vi "创建demo守护脚本文件.vi"(8 "错误输入":errorcluster, 11 "文件路径（使用对话框）":path) -> (0 "错误输出":errorcluster)   [LabVIEW 2016]
panel:
  out "连接的字符串":string
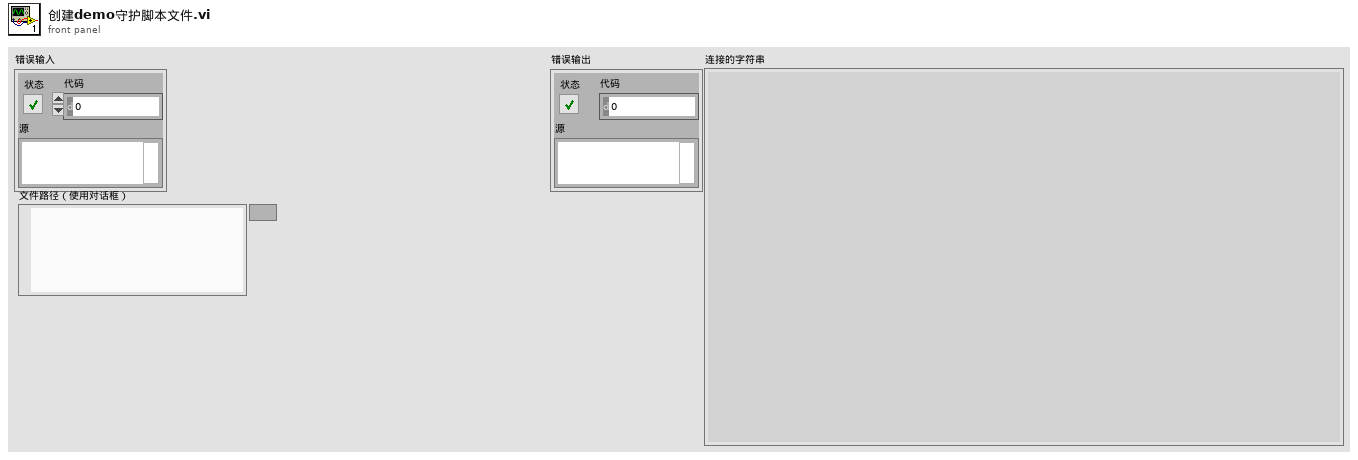
[diagram p1: front panel]
types:
  T1 = enum16{"open", "replace", "create", "open or create", "replace or create", "replace or create with confirmation"}
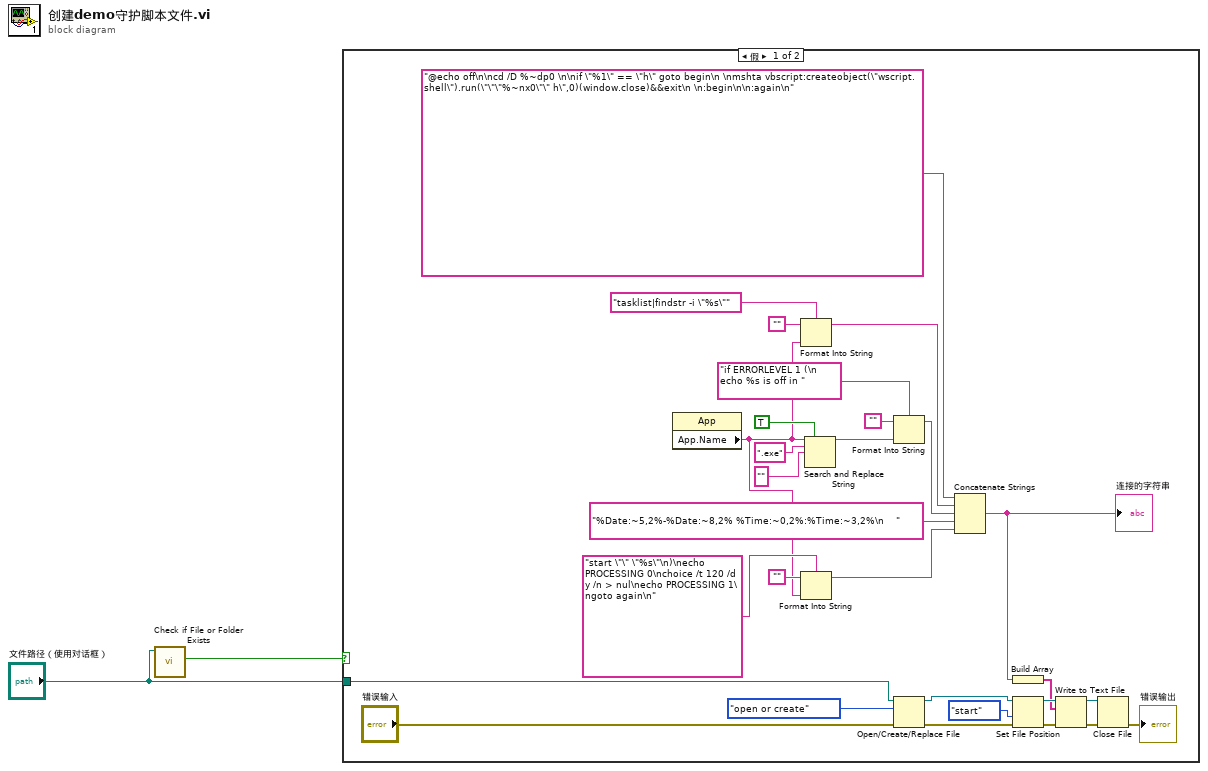
[diagram p0: block diagram]
diagram:
  n1 = call <vilib>:"Check if File or Folder Exists.vi"("path"="文件路径（使用对话框）") -> ("file or folder exists?"=w1:bool)  [unwired: 8 in, 2 out]
  n2 = case shown="假" w1 {
    tunnel: "文件路径（使用对话框）" -> [w3 _]
    frame False {
      n3 = property class="App"() -> ("App.Name"=w6:string)  [unwired: 2 in, 2 out]
      n4 = Format Into String(format string="tasklist|findstr -i \"%s\"", initial string="", w6) -> (resulting string=w10:string)  [unwired: 1 in, 1 out]
      n5 = Format Into String(format string="start \"\" \"%s\"\n)\necho PROCESSING 0\nchoice /t 120 /d y /n > nul\necho PROCESSING 1\ngoto again\n", initial string="", w6) -> (resulting string=w4:string)  [unwired: 1 in, 1 out]
      n6 = Search and Replace String(replace all?=TRUE ("替换全部？(F)"), input string=w6, search string=".exe" ("搜索字符串"), replace string="" ("替换字符串(\"\")")) -> (result string=w12:string)  [unwired: 4 in, 3 out]
      n7 = Format Into String(format string="if ERRORLEVEL 1 (\n    echo %s is off in ", initial string="", w12) -> (resulting string=w9:string)  [unwired: 1 in, 1 out]
      n8 = Open/Create/Replace File(file path (use dialog)=w3, error in="错误输入", operation (0:open)=T1."open or create" ("操作(0:open)")) -> (refnum out=w27:refnum<file>, error out=w28:errorcluster)  [unwired: 3 in, 1 out]
      n9 = Concatenate Strings("@echo off\n\ncd /D %~dp0 \n\nif \"%1\" == \"h\" goto begin\n \nmshta vbscript:createobject(\"wscript.shell\").run(\"\"\"%~nx0\"\" h\",0)(window.close)&&exit\n \n:begin\n\n:again\n", w10, w9, "%Date:~5,2%-%Date:~8,2% %Time:~0,2%:%Time:~3,2%\n    ", w4) -> (w5:string)
      "连接的字符串" <- w5
      n10 = Build Array(w5) -> (w23:string[])
      n11 = Set File Position(refnum=w27, from (0:start)=enum16{"start", "end", "current"}."start" ("自（0:起始）"), error in=w28) -> (refnum out=w29:refnum<file>, error out=w30:errorcluster)  [unwired: 1 in]
      n12 = Write to Text File(file (use dialog)=w29, text=w23, error in=w30) -> (refnum out=w25:refnum<file>, error out=w24:errorcluster)  [unwired: 1 in, 1 out]
      n13 = Close File(refnum=w25, error in=w24) -> (error out=→"错误输出":errorcluster)  [unwired: 1 out]
    }
    frame True {
    }
  }
